vi "NEWDLL Test midiin_main.vi"() -> ()   [LabVIEW 2020]
uses:
  cpp-src/MIDIToLabVIEW/MIDIToLabVIEW/MIDItoLabVIEW.dll
panel:
  out "String":string
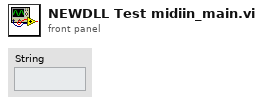
[diagram p1: front panel]
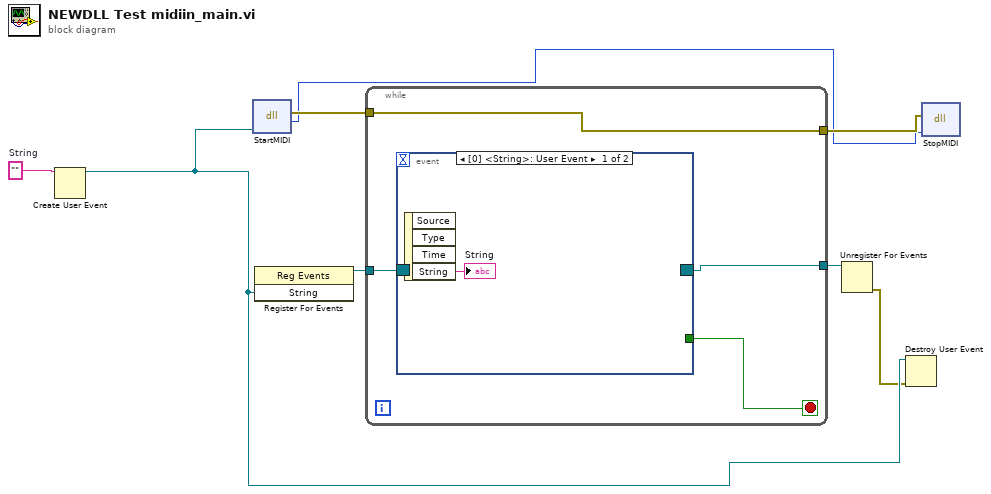
[diagram p0: block diagram]
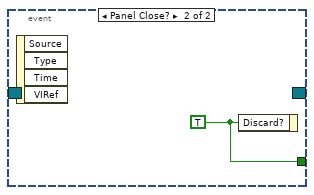
[diagram p2: hidden frame]
diagram:
  w8 = ""  # String
  n1 = Create User Event(user event datatype=w8) -> (user event=w3:refnum<user-event>)  [unwired: 1 in, 1 out]
  n2 = dll-call lib="C:/code/LabVIEW-MIDI/cpp-src/MIDIToLabVIEW/MIDIToLabVIEW/MIDItoLabVIEW.dll" fn="StartMIDI"("event"=w3) -> (error out=w5:errorcluster, "return type"=w1:u64)  [unwired: 4 in, 1 out]
  n3 = register-events(w3) -> (reference out=w7:refnum<event-registration>)  [unwired: 2 in, 1 out]
  n4 = while {
    tunnel: w7 -> [w12]
    tunnel: [w11] -> w6
    tunnel: w5 -> [w11]
    tunnel: [w10] -> w4
    stop <- w9 stop-if-true
    n5 = event shown="[0] <String>: User Event" {
      selector: w12 -> [_ _]
      dyn-events: [_ _] -> w10
      timeout: _ -> [_ _]
      tunnel: [_ w14] -> w9
      event User Event {
        n6 = event-data() -> ("String"=→"String":string)  [unwired: 1 in, 3 out]
      }
      event Panel Close? {
        w14 = TRUE ("Discard?")
        n7 = event-data() -> ()  [unwired: 1 in, 4 out]
        n8 = event-data("Discard?"=w14) -> ()  [unwired: 1 in, 1 out]
      }
    }
  }
  n9 = Unregister For Events(event registration refnum=w4) -> (error out=w2:errorcluster)  [unwired: 1 in]
  n10 = Destroy User Event(user event=w3, error in=w2) -> ()  [unwired: 1 out]
  n11 = dll-call lib="C:/code/LabVIEW-MIDI/cpp-src/MIDIToLabVIEW/MIDIToLabVIEW/MIDItoLabVIEW.dll" fn="StopMIDI"(error in=w6, "arg1"=w1) -> ()  [unwired: 4 in, 2 out]
